vi "SetupSweepAndGetPeak.vi"(6 "Route Names":string[](array[string]), 7 "Cal?":bool=TRUE, 8 "error in (no error)":errorcluster, 9 "Span(Hz)":dbl=26500000000.0, 10 "Center Frequency(Hz)":dbl=13250000000.0, 11 "PwrMtr_RSNRPZ in":refnum<class "PwrMtr_RSNRPZ.lvclass">) -> (0 "error out":errorcluster, 1 "FDelta(hz)":dbl, 2 "Calibrated Amplitude (dBm)":dbl, 3 "PwrMtr_RSNRPZ out":refnum<class "PwrMtr_RSNRPZ.lvclass">)   [LabVIEW 2014, in "PwrMtr_RSNRPZ.lvclass"]
uses:
  PwrMtr_RSNRPZ.lvclass
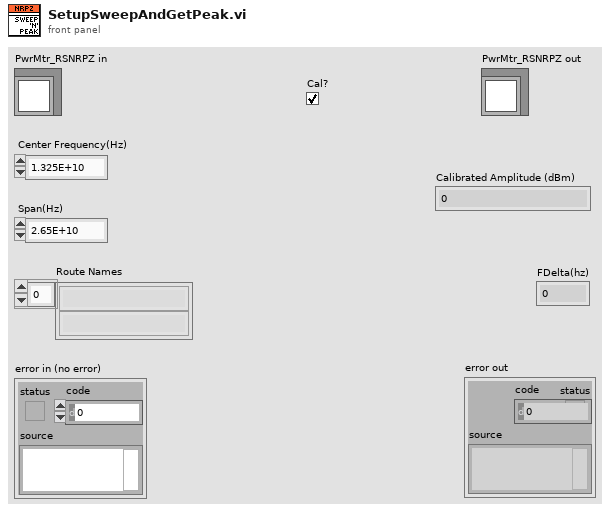
[diagram p1: front panel]
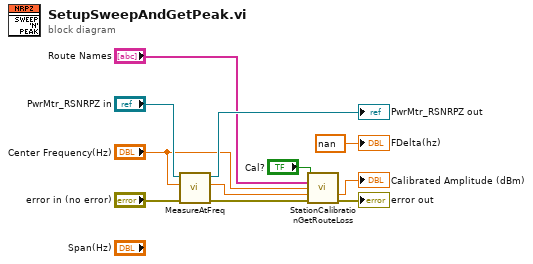
[diagram p0: block diagram]
diagram:
  n1 = call-dynamic "MeasureAtFreq.vi"("error in (no error)"="error in (no error)", "Frequency (Hz)"="Center Frequency(Hz)", "PwrMtr_RSNRPZ in"="PwrMtr_RSNRPZ in") -> ("error out"=w3:errorcluster, "Power (dBm)"=w5:dbl, "PwrMtr_RSNRPZ out"=→"PwrMtr_RSNRPZ out":refnum<class "PwrMtr_RSNRPZ.lvclass">)  [unwired: 6 in]
  n2 = call "StationCalibrationGetRouteLoss.vi"("Calibration Enabled"="Cal?", "Route Names"="Route Names", "Frequency"="Center Frequency(Hz)", "Power Level"=w5, "error in (no error)"=w3) -> ("Adjusted Power Level"=→"Calibrated Amplitude (dBm)":dbl, "error out"=→"error out":errorcluster)  [unwired: 7 in, 2 out]
  "FDelta(hz)" <- nan ("FDelta(hz)")
